vi "LinearFilter.vi"(8 "error in (no error)":errorcluster, 11 "Image Src":T1) -> (0 "error out":errorcluster, 3 "Image":T1(plugin-control))   [LabVIEW 2017]
uses:
  <vilib>/vision/Image Controls.llb/IMAQ Image.ctl
  <vilib>/vision/NI_Vision_Development_Module.lvlib
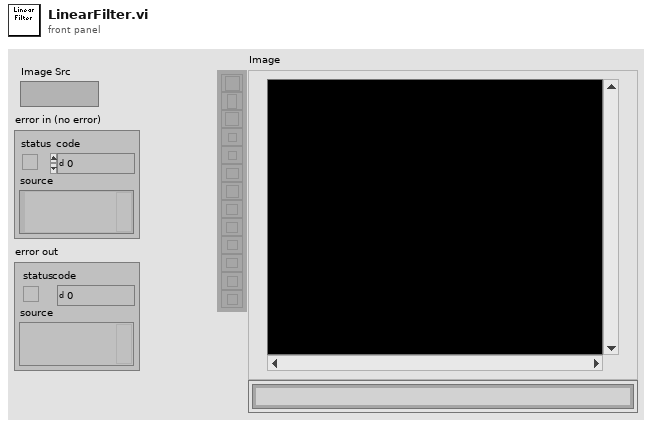
[diagram p1: front panel]
types:
  T1 = typedef "IMAQ Image.ctl" = refnum<image>
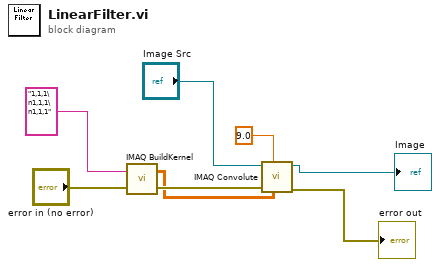
[diagram p0: block diagram]
diagram:
  n1 = call "IMAQ BuildKernel"("Kernel String"="1,1,1\n1,1,1\n1,1,1", "error in (no error)"="error in (no error)") -> ("Kernel"=w5:sgl[][], "error out"=w7:errorcluster)  [unwired: 3 in]
  n2 = call "IMAQ Convolute"("Kernel"=w5, "Divider (kernel sum)"=sgl 9.0, "error in (no error)"=w7, "Image Src"="Image Src") -> ("error out"=→"error out":errorcluster, "Image Dst Out"=→"Image":T1)  [unwired: 6 in]
